vi "TestVoltageDivider.vi"() -> ()   [LabVIEW 2020]
panel:
  in  "Knob":dbl(knob) scale=0.0..10.0
  in  "?":bool
  out "Waveform Chart":dbl(graph)
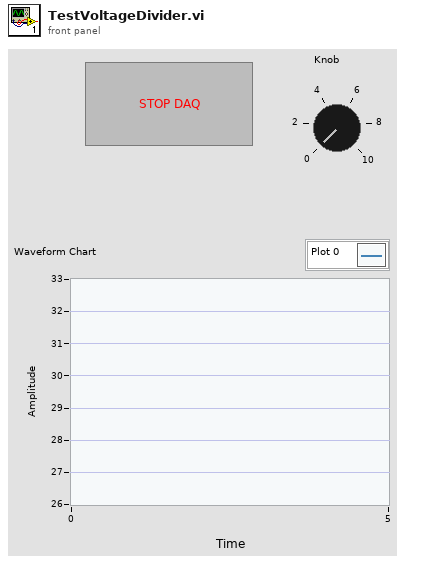
[diagram p1: front panel]
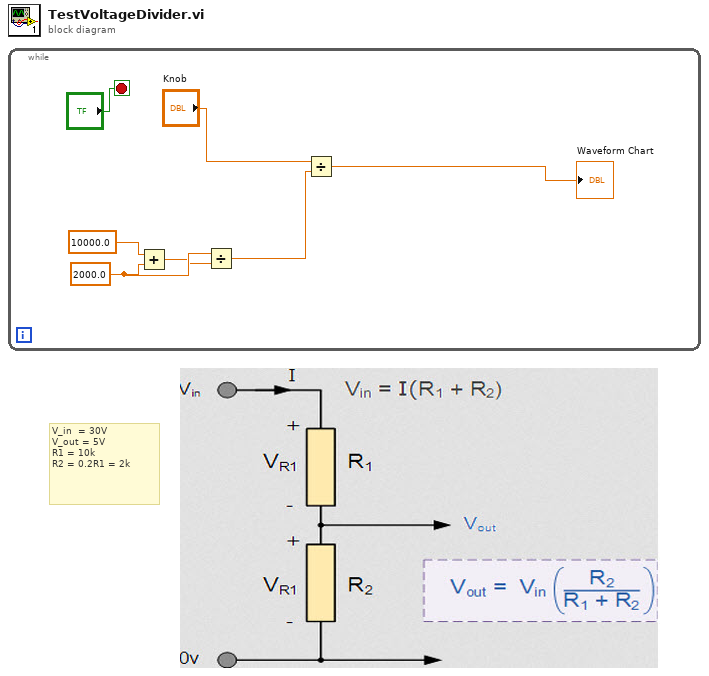
[diagram p0: block diagram]
diagram:
  # "V_in  = 30V \nV_out = 5V\nR1 = 10k \nR2 = 0.2R1 = 2k"
  n1 = while {
    stop <- "?" stop-if-true
    w5 = 2000.0
    n2 = Add(x=10000.0, y=w5) -> (x+y=w4:dbl)
    n3 = Divide(x=w5, y=w4) -> (x/y=w3:dbl)
    n4 = Divide(x="Knob", y=w3) -> (x/y=→"Waveform Chart":dbl)
  }
